vi "compres1.vi"(1 "Numeric":i16, 2 "Array":i16[](array[numeric])) -> (0 "Numeric 2":i16)   [LabVIEW 2010]
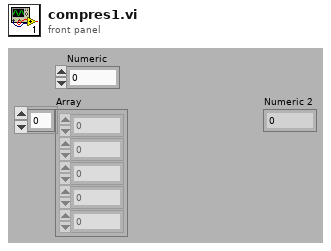
[diagram p1: front panel]
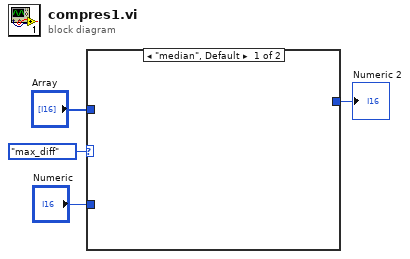
[diagram p0: block diagram]
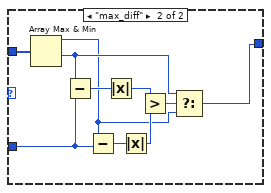
[diagram p2: hidden frame]
diagram:
  n1 = case shown="\"median\", Default" enum16{"median", "max_diff"}."max_diff" {
    tunnel: [_ w5] -> w4
    tunnel: "Array" -> [_ w14]
    tunnel: "Numeric" -> [_ w13]
    frame "median", Default {
    }
    frame "max_diff" {
      n2 = Array Max & Min(array=w14) -> (max value=w6:i16, min value=w7:i16)  [unwired: 2 out]
      n3 = Subtract(x=w7, y=w13) -> (x-y=w11:i16)
      n4 = Subtract(x=w6, y=w13) -> (x-y=w12:i16)
      n5 = Absolute Value(x=w11) -> (abs(x)=w10:i16)
      n6 = Absolute Value(x=w12) -> (abs(x)=w9:i16)
      n7 = Greater?(x=w10, y=w9) -> (0:w8:bool)
      n8 = Select(t=w7, s=w8, f=w6) -> (s? t:f=w5:i16)
    }
  }
  "Numeric 2" <- w4
